vi "Initialize GV.vi"() -> ()   [LabVIEW 2019, in "Initialize.lvlib"]
uses:
  Initialize.lvlib
panel:
  in  "Folder Path":path
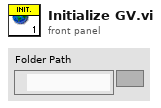
[diagram p1: front panel]
diagram:
